vi "DriveDistanceY.vi"(1 "Parameter String":string, 2 "Reinit":bool) -> (0 "Increment":bool)   [LabVIEW 2019]
uses:
  dsinstructions.vi
  sensors.vi
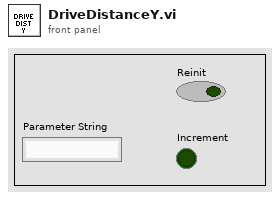
[diagram p1: front panel]
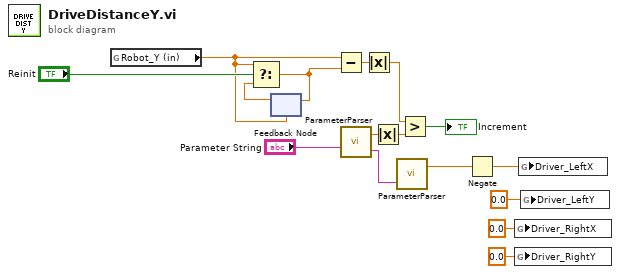
[diagram p0: block diagram]
diagram:
  n1 = global read "sensors.vi" "Robot_Y (in)"() -> (w13:dbl)
  n2 = feedback #1(w13) -> (w15:dbl)
  n3 = Select(t=w13, s="Reinit", f=w15) -> (s? t:f=w12:dbl)
  n4 = feedback-in #1(w12) -> ()
  n5 = Subtract(x=w13, y=w12) -> (x-y=w11:dbl)
  n6 = call "ParameterParser.vi"("Parameter String"="Parameter String") -> ("Remaining Parameter String"=w7:string, "Parameter"=w8:dbl)  [unwired: 1 in]
  n7 = Absolute Value(x=w11) -> (abs(x)=w2:dbl)
  n8 = Absolute Value(x=w8) -> (abs(x)=w1:dbl)
  n9 = call "ParameterParser.vi"("Parameter String"=w7) -> ("Parameter"=w6:dbl)  [unwired: 1 in, 1 out]
  n10 = Greater?(x=w2, y=w1) -> (0:→"Increment":bool)
  n11 = Negate(x=w6) -> (-x=w3:dbl)
  n12 = global write "dsinstructions.vi" "Driver_RightX"(0.0 ("Driver_RightX")) -> ()
  n13 = global write "dsinstructions.vi" "Driver_RightY"(0.0 ("Driver_RightX")) -> ()
  n14 = global write "dsinstructions.vi" "Driver_LeftX"(w3) -> ()
  n15 = global write "dsinstructions.vi" "Driver_LeftY"(0.0 ("Driver_RightX")) -> ()
